vi "Post Process Data Averaging.vi"(0 "pInputImage":i32, 1 "iAveragingFilterMode":i32, 2 "iWidth":i32, 3 "iAveragingFactor":i32, 5 "pOutputImage":i32, 7 "iOutputBufferSize":i32, 9 "iNumImages":i32, 12 "iHeight":i32, 13 "iFrameCount":i32) -> (4 "pInputImage out":i32, 6 "pOutputImage out":i32, 8 "function return":u32)   [LabVIEW 2018, in "Copy of Andor SDK.lvlib"]
doc: "EXPNETTYPE unsigned int WINAPI PostProcessDataAveraging(at_32 * pInputImage, at_32 * pOutputImage, int iOutputBufferSize, int iNumImages, int iAveragingFilterMode, int iHeight, int iWidth, int iFrameCount, int iAveragingFactor);"
uses:
  Copy of Andor SDK.lvlib
  <userlib>/Andor SDK/ATMCD32D.dll
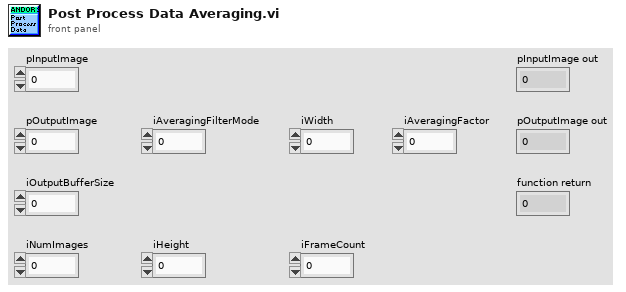
[diagram p1: front panel]
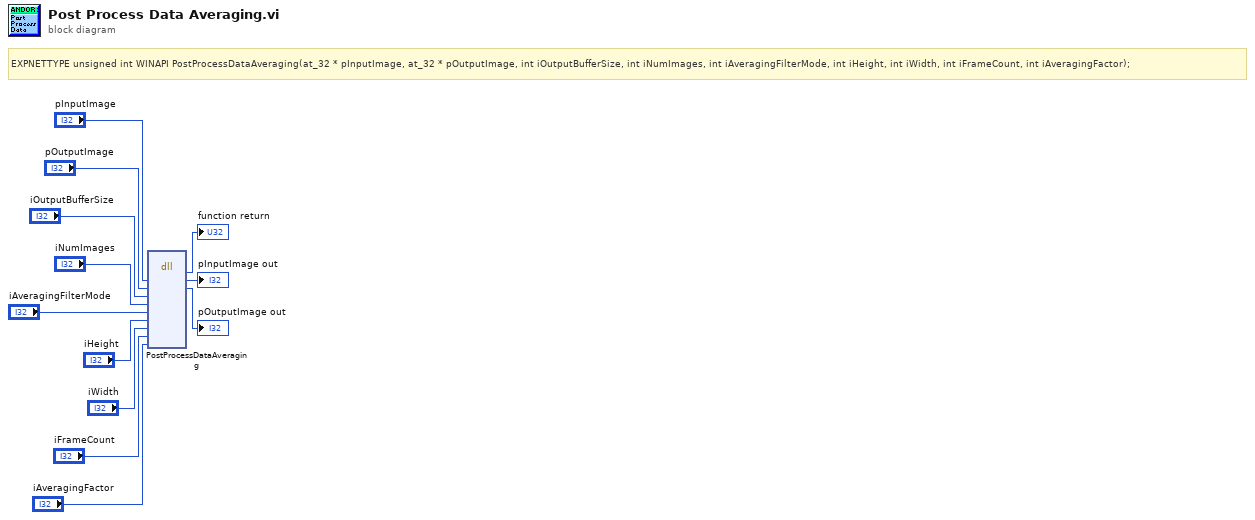
[diagram p0: block diagram]
diagram:
  # "EXPNETTYPE unsigned int WINAPI PostProcessDataAveraging(at_32 * pInputImage, at_32 * pOutputImage, int iOutputBufferSize, int iNumImages, int iAveragingFilterMode, int iHeight, int iWidth, int iFrameCount, int iAveragingFactor);"
  n1 = dll-call lib="C:/Program Files (x86)/National Instruments/LabVIEW 2018/user.lib/Andor SDK/ATMCD32D.*" fn="PostProcessDataAveraging"("pInputImage"="pInputImage", "pOutputImage"="pOutputImage", "iOutputBufferSize"="iOutputBufferSize", "iNumImages"="iNumImages", "iAveragingFilterMode"="iAveragingFilterMode", "iHeight"="iHeight", "iWidth"="iWidth", "iFrameCount"="iFrameCount", "iAveragingFactor"="iAveragingFactor") -> (→"function return":u32, "pInputImage"=→"pInputImage out":i32, "pOutputImage"=→"pOutputImage out":i32)  [unwired: 10 in, 2 out]
